vi "Parse Serial Channel String.vi"(11 "Serial Channel String":string) -> (2 "Channel Number":i32, 3 "Serial Channel Type":T1(ring))   [LabVIEW 2025, in "I2C Bus Monitor.lvclass"]
uses:
  I2C Bus Monitor.lvclass
  <vilib>/Utility/error.llb/Trim Whitespace One-Sided.vi
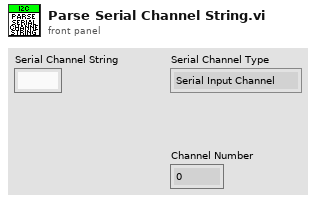
[diagram p1: front panel]
types:
  T1 = enum16{"Serial Input Channel", "Serial Output Channel", "Unknown Channel Type"}
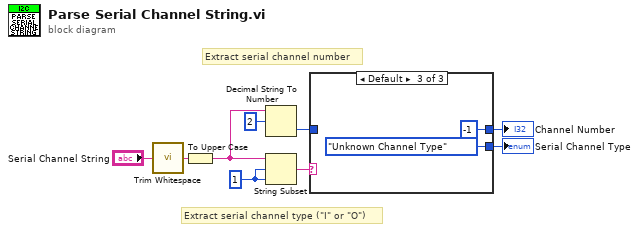
[diagram p0: block diagram]
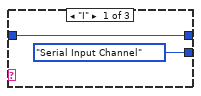
[diagram p2: hidden frame]
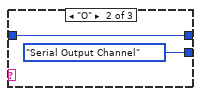
[diagram p3: hidden frame]
diagram:
  w5 = 1 ("length (rest)")
  # "Extract serial channel type (\"I\" or \"O\")"
  # "Extract serial channel number"
  n1 = call <vilib>:"Trim Whitespace.vi"("string"="Serial Channel String") -> ("trimmed string"=w3:string)  [unwired: 1 in]
  n2 = To Upper Case(1:w3) -> (0:w2:string)
  n3 = Decimal String To Number(string=w2, offset=2) -> (number=w7:i32)  [unwired: 1 in, 1 out]
  n4 = String Subset(string=w2, offset (0)=w5, length (rest)=w5) -> (substring=w9:string)
  n5 = case shown="Default" w9 {
    tunnel: [T1."Serial Input Channel" T1."Serial Output Channel" T1."Unknown Channel Type"] -> w8
    tunnel: w7 -> [w10 w12 _]
    tunnel: [w10 w12 -1] -> w6
    frame "I" {
    }
    frame "O" {
    }
    frame Default {
    }
  }
  "Serial Channel Type" <- w8
  "Channel Number" <- w6
